vi "Array of Variants to JSON Object.vi"(5 "enable LabVIEW extensions? (T)":bool=TRUE, 6 "Pretty Print?":bool, 9 "error in (no error)":errorcluster, 10 "Names":string[](array[string]), 11 "Array":variant[](array[variant])) -> (1 "error out":errorcluster, 3 "<JSON>":string)   [LabVIEW 2017, in "JSONtext.lvlib"]
doc: "Flatten an Array of Variants into a JSON Object. If item names are not supplied, they will be taken from the data name in the Variants.\n\nStrings or Arrays of strings marked with a leading \"<JSON>\" tag in their name (including inside clusters) are treated as already being valid JSON. Strings not marked as <JSON> are quoted and escaped as a JSON String."
uses:
  JSONtext.lvlib
  <vilib>/Utility/Data Type/NI_Data Type.lvlib
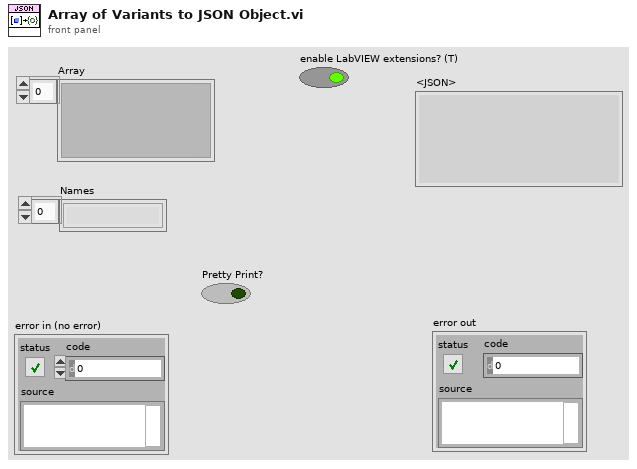
[diagram p1: front panel]
types:
  T1 = typedef "NI_Data Type.lvlib/Data Type.ctl" = enum8{"Invalid Type", "Void", "I8", "I16", "I32", "I64", "U8", "U16", "U32", "U64", "Single Float", "Double Float", "Extended Float", "Single Complex", "Double Complex", "Extended Complex", "Enum U8", "Enum U16", "Enum U32", "Enum U64", "Single Float With Unit", "Double Float With Unit", "Extended Float With Unit", "Single Complex with Unit", "Double Complex with Unit", "Extended Complex with Unit", "Boolean", "String", "Path", "Picture", "Tag", "Array", "Cluster", "Variant", "LV Variant", "Waveform", "Timestamp", "Digital Waveform", "Digital Data", "ExpressData", "Refnum", "External Data", "VI", "Poly VI", "LabVIEW Class Instance", "Fixed Point"}
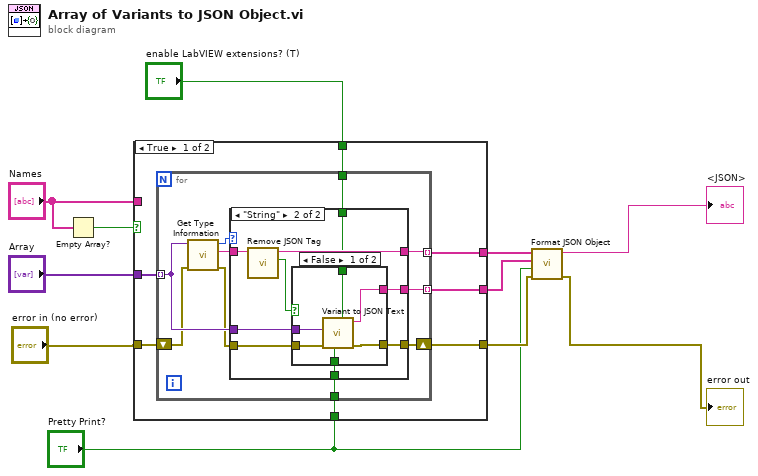
[diagram p0: block diagram]
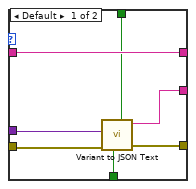
[diagram p2: hidden frame]
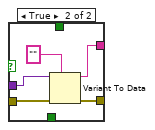
[diagram p3: hidden frame]
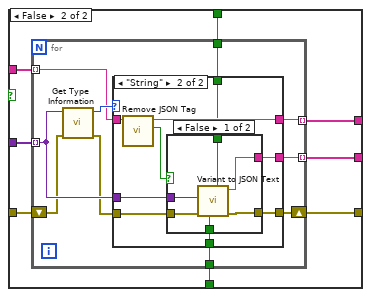
[diagram p4: hidden frame]
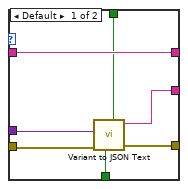
[diagram p5: hidden frame]
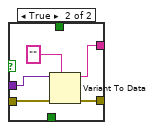
[diagram p6: hidden frame]
diagram:
  n1 = Empty Array?(array="Names") -> (empty?=w4:bool)
  n2 = case shown="True" w4 {
    tunnel: [w18 w63] -> w10
    tunnel: [w17 w62] -> w8
    tunnel: [w16 w61] -> w7
    tunnel: "error in (no error)" -> [w15 w60]
    tunnel: "Array" -> [w14 w59]
    tunnel: "Names" -> [_ w56]
    tunnel: "Pretty Print?" -> [w13 w58]
    tunnel: "enable LabVIEW extensions? (T)" -> [w12 w57]
    frame True {
      n3 = for {
        shift-right: [w26] -> w18
        shift-left: w15 -> [w20]
        tunnel: w14 -> [w28] mode=indexing
        tunnel: [w22] -> w17 mode=indexing
        tunnel: [w25] -> w16 mode=indexing
        tunnel: w13 -> [w24]
        tunnel: w12 -> [w23]
        n4 = call <vilib>:"Get Type Information.vi"("error in (no error)"=w20, "Variant"=w28) -> ("error out"=w19:errorcluster, "Name"=w27:string, "Type"=w21:T1)  [unwired: 5 in, 2 out]
        n5 = case shown="\"String\"" w21 {
          tunnel: w28 -> [w30 w44]
          tunnel: w27 -> [w35 w43]
          tunnel: w19 -> [w31 w42]
          tunnel: [w34 w41] -> w26
          tunnel: [w35 w40] -> w25
          tunnel: w24 -> [w32 w39]
          tunnel: w23 -> [w33 w38]
          tunnel: [w29 w37] -> w22
          frame Default {
            n6 = call "Variant to JSON Text.vi"("enable LabVIEW extensions? (T)"=w33, "Pretty Print?"=w32, "error in (no error)"=w31, "Variant"=w30) -> ("error out"=w34:errorcluster, "<JSON>"=w29:string)  [unwired: 5 in, 1 out]
          }
          frame "String" {
            n7 = call "Remove JSON Tag.vi"("Name"=w43) -> ("tagged as JSON text"=w36:bool, "Name (tag stripped)"=w40:string)  [unwired: 9 in]
            n8 = case shown="False" w36 {
              tunnel: w44 -> [w50 w53]
              tunnel: w42 -> [w49 w54]
              tunnel: [w48 w55] -> w41
              tunnel: w39 -> [w47 _]
              tunnel: w38 -> [w46 _]
              tunnel: [w45 w51] -> w37
              frame False {
                n9 = call "Variant to JSON Text.vi"("enable LabVIEW extensions? (T)"=w46, "Pretty Print?"=w47, "error in (no error)"=w49, "Variant"=w50) -> ("error out"=w48:errorcluster, "<JSON>"=w45:string)  [unwired: 5 in, 1 out]
              }
              frame True {
                n10 = Variant To Data(error in=w54, type="", Variant=w53) -> (data=w51:string, error out=w55:errorcluster)
              }
            }
          }
        }
      }
    }
    frame False {
      n11 = for {
        shift-right: [w72] -> w63
        shift-left: w60 -> [w66]
        tunnel: w59 -> [w73] mode=indexing
        tunnel: [w68] -> w62 mode=indexing
        tunnel: [w71] -> w61 mode=indexing
        tunnel: w58 -> [w70]
        tunnel: w57 -> [w69]
        tunnel: w56 -> [w64] mode=indexing
        n12 = call <vilib>:"Get Type Information.vi"("error in (no error)"=w66, "Variant"=w73) -> ("error out"=w65:errorcluster, "Type"=w67:T1)  [unwired: 5 in, 3 out]
        n13 = case shown="\"String\"" w67 {
          tunnel: w73 -> [w75 w89]
          tunnel: w64 -> [w80 w88]
          tunnel: w65 -> [w76 w87]
          tunnel: [w79 w86] -> w72
          tunnel: [w80 w85] -> w71
          tunnel: w70 -> [w77 w84]
          tunnel: w69 -> [w78 w83]
          tunnel: [w74 w82] -> w68
          frame Default {
            n14 = call "Variant to JSON Text.vi"("enable LabVIEW extensions? (T)"=w78, "Pretty Print?"=w77, "error in (no error)"=w76, "Variant"=w75) -> ("error out"=w79:errorcluster, "<JSON>"=w74:string)  [unwired: 5 in, 1 out]
          }
          frame "String" {
            n15 = call "Remove JSON Tag.vi"("Name"=w88) -> ("tagged as JSON text"=w81:bool, "Name (tag stripped)"=w85:string)  [unwired: 9 in]
            n16 = case shown="False" w81 {
              tunnel: w89 -> [w95 w98]
              tunnel: w87 -> [w94 w99]
              tunnel: [w93 w100] -> w86
              tunnel: w84 -> [w92 _]
              tunnel: w83 -> [w91 _]
              tunnel: [w90 w96] -> w82
              frame False {
                n17 = call "Variant to JSON Text.vi"("enable LabVIEW extensions? (T)"=w91, "Pretty Print?"=w92, "error in (no error)"=w94, "Variant"=w95) -> ("error out"=w93:errorcluster, "<JSON>"=w90:string)  [unwired: 5 in, 1 out]
              }
              frame True {
                n18 = Variant To Data(error in=w99, type="", Variant=w98) -> (data=w96:string, error out=w100:errorcluster)
              }
            }
          }
        }
      }
    }
  }
  n19 = call "Format JSON Object.vi"("error in (no error)"=w10, "Pretty Print?"="Pretty Print?", "JSON elements"=w8, "Names"=w7) -> ("error out"=→"error out":errorcluster, "JSON Object Text out"=→"<JSON>":string)  [unwired: 6 in]
